vi "Trying_Arduino_Control_Motor.vi"() -> ()   [LabVIEW 2012]
uses:
  <vilib>/NXT/Block Support/HWPage.SensorType.ctl
  <vilib>/NXT/Block Support/HWPage.SensorMode.ctl
  <vilib>/NXT/Block Support/NXT_InputPort.ctl
  <vilib>/NXT/Subs/MotorOutput.ctl
  <vilib>/NXT/Dual Mode Library/Sensors/i2c_sensors.vi
  <vilib>/NXT/Dual Mode Library/Display/drawText.vi
  <vilib>/NXT/Dual Mode Library/Waits/Wait_NXTFlag.vi
  <vilib>/NXT/Dual Mode Library/Advanced/NXTFlag_Assign.vi
panel:
  out "Motor":dbl(knob) scale=0.0..360.0
  out "Motor":dbl
  out "Motor":dbl
  out "Motor":dbl(knob) scale=0.0..360.0
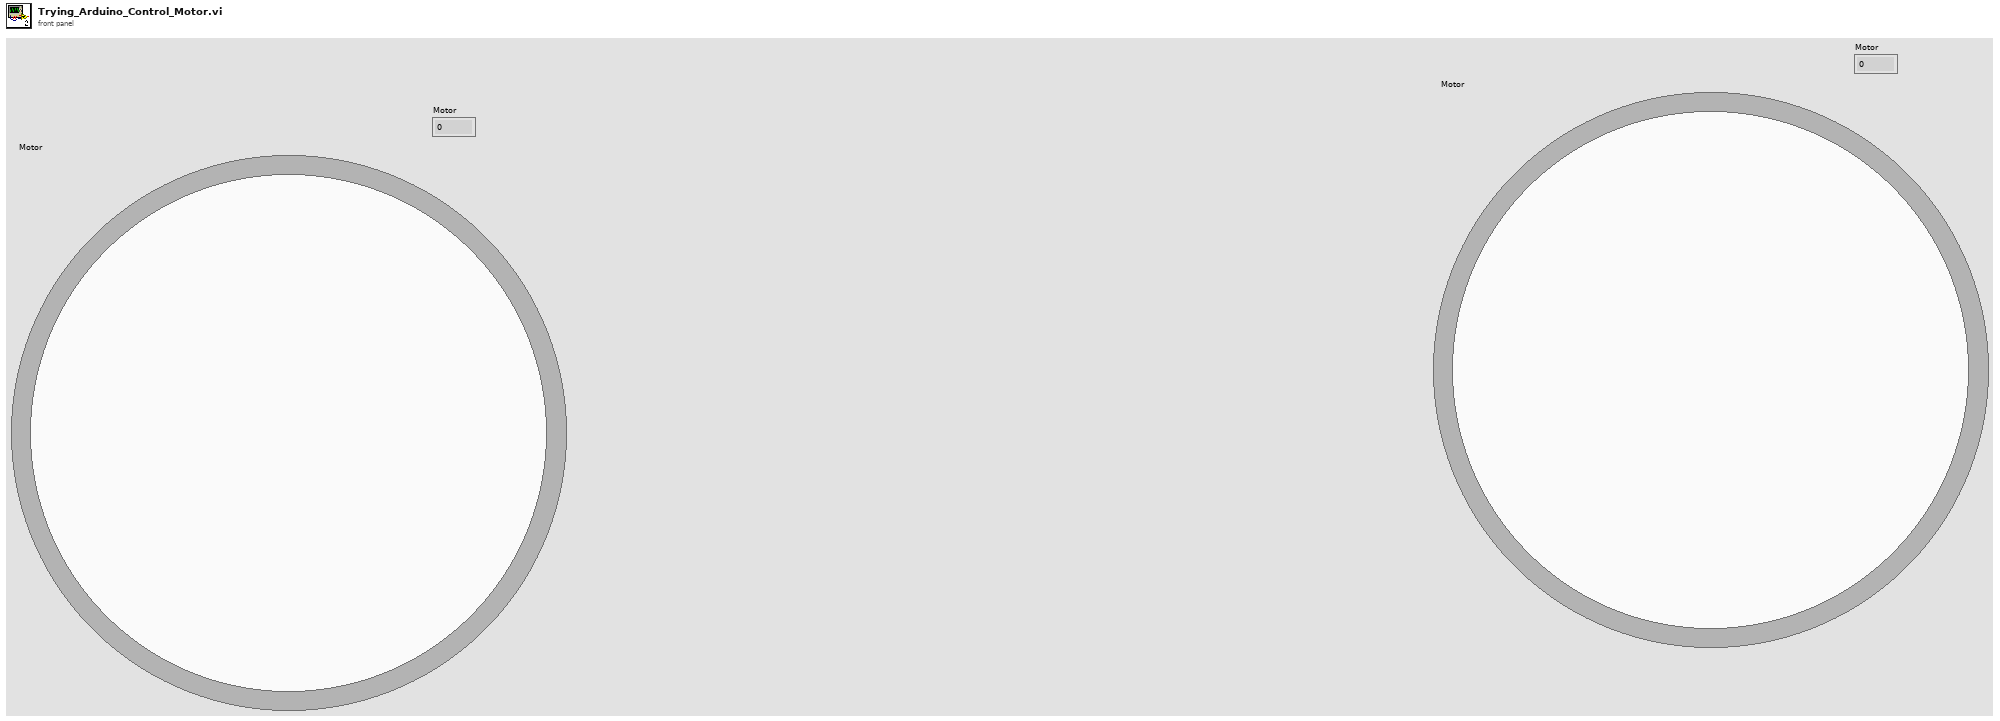
[diagram p1: front panel]
types:
  T1 = typedef "MotorOutput.ctl" = u8
  T2 = typedef "NXT_InputPort.ctl" = u8
  T3 = typedef "HWPage.SensorType.ctl" = u8
  T4 = typedef "HWPage.SensorMode.ctl" = u8
  T5 = typedef "LVHSConnector.ctl" = cluster{"Hardware":string, "Flattened String":string}
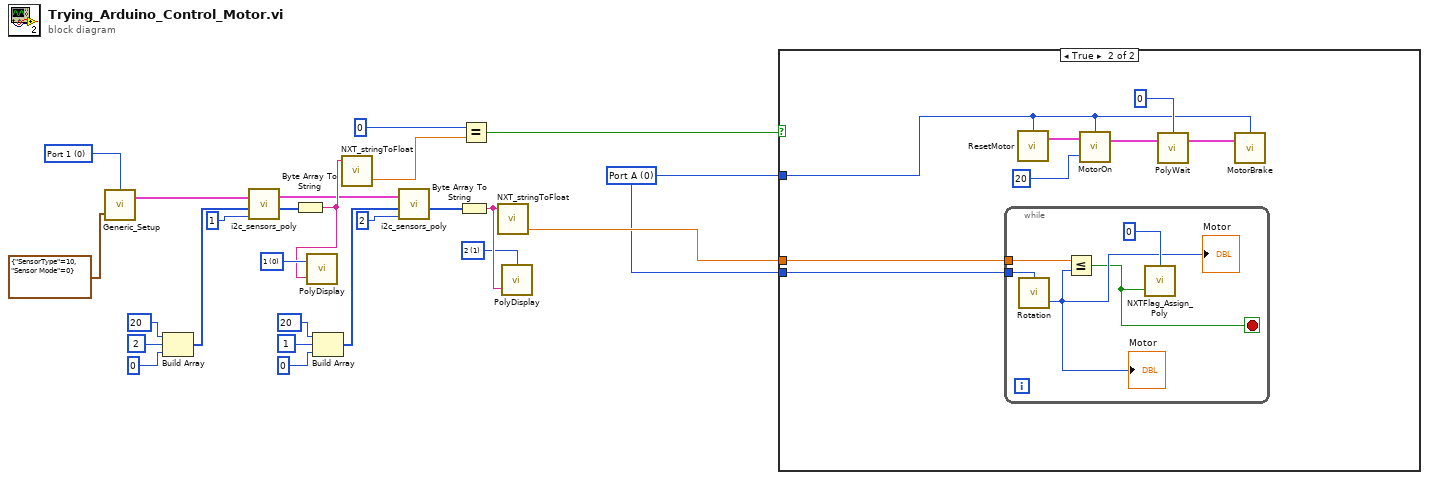
[diagram p0: block diagram]
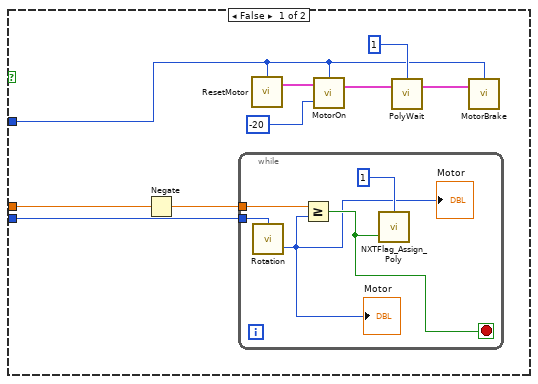
[diagram p2: hidden frame]
diagram:
  w5 = i16 0 items=["1", "2", "3", "4", "5", "6", "7", "8"] ("Line")
  w22 = i16 1 items=["1", "2", "3", "4", "5", "6", "7", "8"] ("Line")
  w8 = T1 0 items=["Port A"=0, "Port B"=1, "Port C"=2, "Ports A & B"=4, "Ports A & C"=5, "Ports B & C"=6, "All Ports"=3] ("Port (All Ports)")
  w24 = T2 0 items=["Port 1", "Port 2", "Port 3", "Port 4"] ("Port")
  n1 = call <vilib>:"Generic_Setup.vi"("Sensor Setup"=cluster{"SensorType":T3, "Sensor Mode":T4} {"SensorType"=10, "Sensor Mode"=0}, "Port"=w24) -> ("NXT"=w10:T5)  [unwired: 1 in, 1 out]
  n2 = Build Array(u8 20, 2, 0 ("element")) -> (w14:i32[])
  n3 = call-poly <vilib>:"i2c_sensors_poly.vi"("Return Length"=u8 1, "Bytes to Write"=w14, "NXT"=w10) -> ("Bytes read"=w7:u8[], "NXT"=w1:T5)  [unwired: 2 in, 1 out]
  n4 = Byte Array To String(unsigned byte array=w7) -> (string=w4:string)
  n5 = call-poly <vilib>:"PolyDisplay.vi"("Text"=w4, "Line"=w5) -> ()  [unwired: 2 in, 1 out]
  n6 = Build Array(u8 20, 1, 0 ("element")) -> (w19:i32[])
  n7 = call <vilib>:"NXT_stringToFloat.vi"("string"=w4) -> ("number"=w3:sgl)  [unwired: 2 in, 1 out]
  n8 = call-poly <vilib>:"i2c_sensors_poly.vi"("Return Length"=u8 2, "Bytes to Write"=w19, "NXT"=w1) -> ("Bytes read"=w20:u8[])  [unwired: 2 in, 2 out]
  n9 = Byte Array To String(unsigned byte array=w20) -> (string=w23:string)
  n10 = Equal?(x=0, y=w3) -> (x = y?=w6:bool)
  n11 = call <vilib>:"NXT_stringToFloat.vi"("string"=w23) -> ("number"=w9:sgl)  [unwired: 2 in, 1 out]
  n12 = call-poly <vilib>:"PolyDisplay.vi"("Text"=w23, "Line"=w22) -> ()  [unwired: 2 in, 1 out]
  n13 = case shown="True" w6 {
    tunnel: w8 -> [w26 w42]
    tunnel: w9 -> [w28 w41]
    tunnel: w8 -> [w29 w40]
    frame False {
      n14 = Negate(x=w28) -> (-x=w27:sgl)
      n15 = while {
        tunnel: w27 -> [w36]
        tunnel: w26 -> [w38]
        stop <- w37 stop-if-true
        n16 = call <vilib>:"Rotation.vi"("Port (Port A)"=w38) -> ("Angle of Rotation"=w35:i32)  [unwired: 2 in, 1 out]
        "Motor" <- w35
        "Motor" <- w35
        n17 = Greater Or Equal?(x=w36, y=w35) -> (x >= y?=w37:bool)
        n18 = call-poly <vilib>:"NXTFlag_Assign_Poly.vi"("Flag State"=w37, "NXT Flag Number"=u8 1 ("Return Length")) -> ()  [unwired: 2 in, 1 out]
      }
      n19 = call <vilib>:"ResetMotor.vi"("Port (All Ports)"=w29) -> ("NXT"=w30:T5)  [unwired: 3 in]
      n20 = call <vilib>:"MotorOn.vi"("Power (75)"=-20, "NXT"=w30, "Output Port (All Ports)"=w29) -> ("NXT"=w32:T5)  [unwired: 1 in]
      n21 = call-poly <vilib>:"PolyWait.vi"("NXT"=w32, "NXT Flag Number"=u8 1 ("Return Length")) -> ("NXT"=w33:T5)  [unwired: 2 in]
      n22 = call <vilib>:"MotorBrake.vi"("NXT"=w33, "Port (All Ports)"=w29) -> ()  [unwired: 2 in, 1 out]
    }
    frame True {
      n23 = while {
        tunnel: w41 -> [w50]
        tunnel: w42 -> [w51]
        stop <- w48 stop-if-true
        n24 = call <vilib>:"Rotation.vi"("Port (Port A)"=w51) -> ("Angle of Rotation"=w49:i32)  [unwired: 2 in, 1 out]
        "Motor" <- w49
        "Motor" <- w49
        n25 = Less Or Equal?(x=w50, y=w49) -> (x <= y?=w48:bool)
        n26 = call-poly <vilib>:"NXTFlag_Assign_Poly.vi"("Flag State"=w48, "NXT Flag Number"=u8 0 ("Return Length")) -> ()  [unwired: 2 in, 1 out]
      }
      n27 = call <vilib>:"ResetMotor.vi"("Port (All Ports)"=w40) -> ("NXT"=w43:T5)  [unwired: 3 in]
      n28 = call <vilib>:"MotorOn.vi"("Power (75)"=20, "NXT"=w43, "Output Port (All Ports)"=w40) -> ("NXT"=w45:T5)  [unwired: 1 in]
      n29 = call-poly <vilib>:"PolyWait.vi"("NXT"=w45, "NXT Flag Number"=u8 0 ("Return Length")) -> ("NXT"=w46:T5)  [unwired: 2 in]
      n30 = call <vilib>:"MotorBrake.vi"("NXT"=w46, "Port (All Ports)"=w40) -> ()  [unwired: 2 in, 1 out]
    }
  }
